vi "LineScanController.vi"() -> ()   [LabVIEW 2022 SP3]
uses:
  Control_LineScanCounterAE.ctl
panel:
  out "Linescan active":bool
  in  "Halt program":bool
  in  "Stop linescan":bool
  in  "Start linescan":bool
  in  "# of Accumulations":i32=2
  in  "# of Points":i32=2 min=1 max=1000
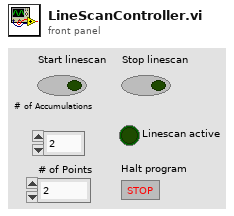
[diagram p1: front panel]
types:
  T1 = enum16{"Start linescan", "Sit Idle", "Stop linescan"}
  T2 = typedef "Control_LineScanCounterAE.ctl" = enum16{"Initialize", "Attach indicators", "Increment Point", "Query", "Do Finish Point", "Acknowledge line", "Deactivate"}
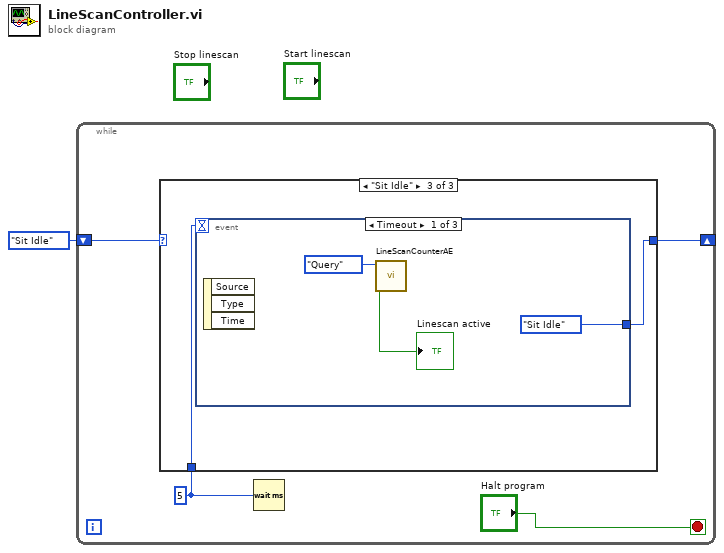
[diagram p0: block diagram]
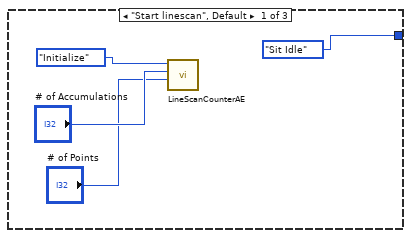
[diagram p2: hidden frame]
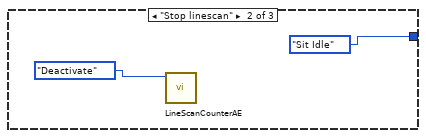
[diagram p3: hidden frame]
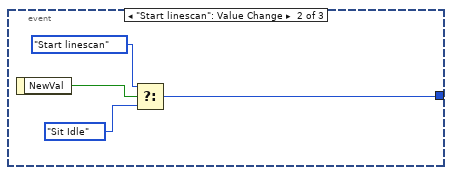
[diagram p4: hidden frame]
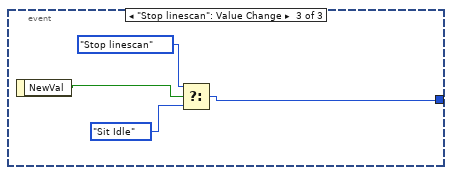
[diagram p5: hidden frame]
diagram:
  n1 = while {
    shift-right: [w4] -> _
    shift-left: T1."Sit Idle" -> [w5]
    stop <- "Halt program" stop-if-true
    w2 = 5
    n2 = case shown="\"Sit Idle\"" w5 {
      tunnel: [T1."Sit Idle" T1."Sit Idle" w12] -> w4
      tunnel: w2 -> [_ _ w13]
      frame "Start linescan", Default {
        n3 = call "LineScanCounterAE.vi"("Number of points"="# of Points", "Accumulate to #"="# of Accumulations", "Task"=Control_LineScanCounterAE."Initialize" ("Enum")) -> ()  [unwired: 2 in, 7 out]
      }
      frame "Stop linescan" {
        n4 = call "LineScanCounterAE.vi"("Task"=Control_LineScanCounterAE."Deactivate" ("Enum")) -> ()  [unwired: 4 in, 7 out]
      }
      frame "Sit Idle" {
        n5 = event shown="[0] Timeout" {
          selector: _ -> [_ _ _]
          dyn-events: _ -> [_ _ _]
          timeout: w13 -> [_ _ _]
          tunnel: [T1."Sit Idle" w17 w21] -> w12
          event Timeout {
            n6 = event-data() -> ()  [unwired: 1 in, 3 out]
            n7 = call "LineScanCounterAE.vi"("Task"=Control_LineScanCounterAE."Query" ("Enum")) -> ("Active"=→"Linescan active":bool)  [unwired: 4 in, 6 out]
          }
          event "Start linescan": Value Change {
            n8 = event-data() -> ("NewVal"=w20:bool)  [unwired: 1 in]
            n9 = Select(t=T1."Start linescan", s=w20, f=T1."Sit Idle") -> (s? t:f=w17:T1)
          }
          event "Stop linescan": Value Change {
            n10 = event-data() -> ("NewVal"=w22:bool)  [unwired: 1 in]
            n11 = Select(t=T1."Stop linescan", s=w22, f=T1."Sit Idle") -> (s? t:f=w21:T1)
          }
        }
      }
    }
    n12 = Wait (ms)(milliseconds to wait=w2) -> ()  [unwired: 1 out]
  }
